vi "LAST 2.vi"() -> ()   [LabVIEW 2020]
uses:
  <vilib>/Instr/_visa.llb/VISA Configure Serial Port (Instr).vi
  <vilib>/measure/matone.llb/Extract Single Tone Information N Chan.vi
  <vilib>/measure/NI_MAPro.lvlib
panel:
  out "Filtered":dynamicdata(graph)
  out ".not. x?":bool
  out "?":dbl format="%#_4g"
  out "?":bool
  out "Gas level":dbl(knob) scale=0.0..2.0
  out "Buzzer":bool
  out "?":bool
  out "?":dbl
  out "Capacitor temperature":dbl(knob) scale=0.0..50.0
  out "Corrected Power Factor":dbl format="%#_4g"
  out "Active power(P)":dbl
  out "Reactive power(Q)":dbl
  out "Apperant power (S)":dbl
  out "Cap B":bool
  out "Cap A":bool
  out "Load Power Factor":dbl format="%#_4g"
  out "Calibearted\nPhase Angle (Radians)":dbl
  out "Calibearted\nPhase Angle (degrees)":dbl
  out "Real \nphase angle":dbl
  out "Current \nphase angle":dbl
  out "Voltage \nphase angle":dbl
  out "Cooling fan":bool
  in  "Virtual phase angle shifter":dbl(slide) scale=0.0..50.0
  in  "VISA resource name":refnum<visa-resource-name>
  in  "baud rate (9600)":u32=9600
  in  "Stop":bool
  # "Smart APFC Panel Control Dashboard"
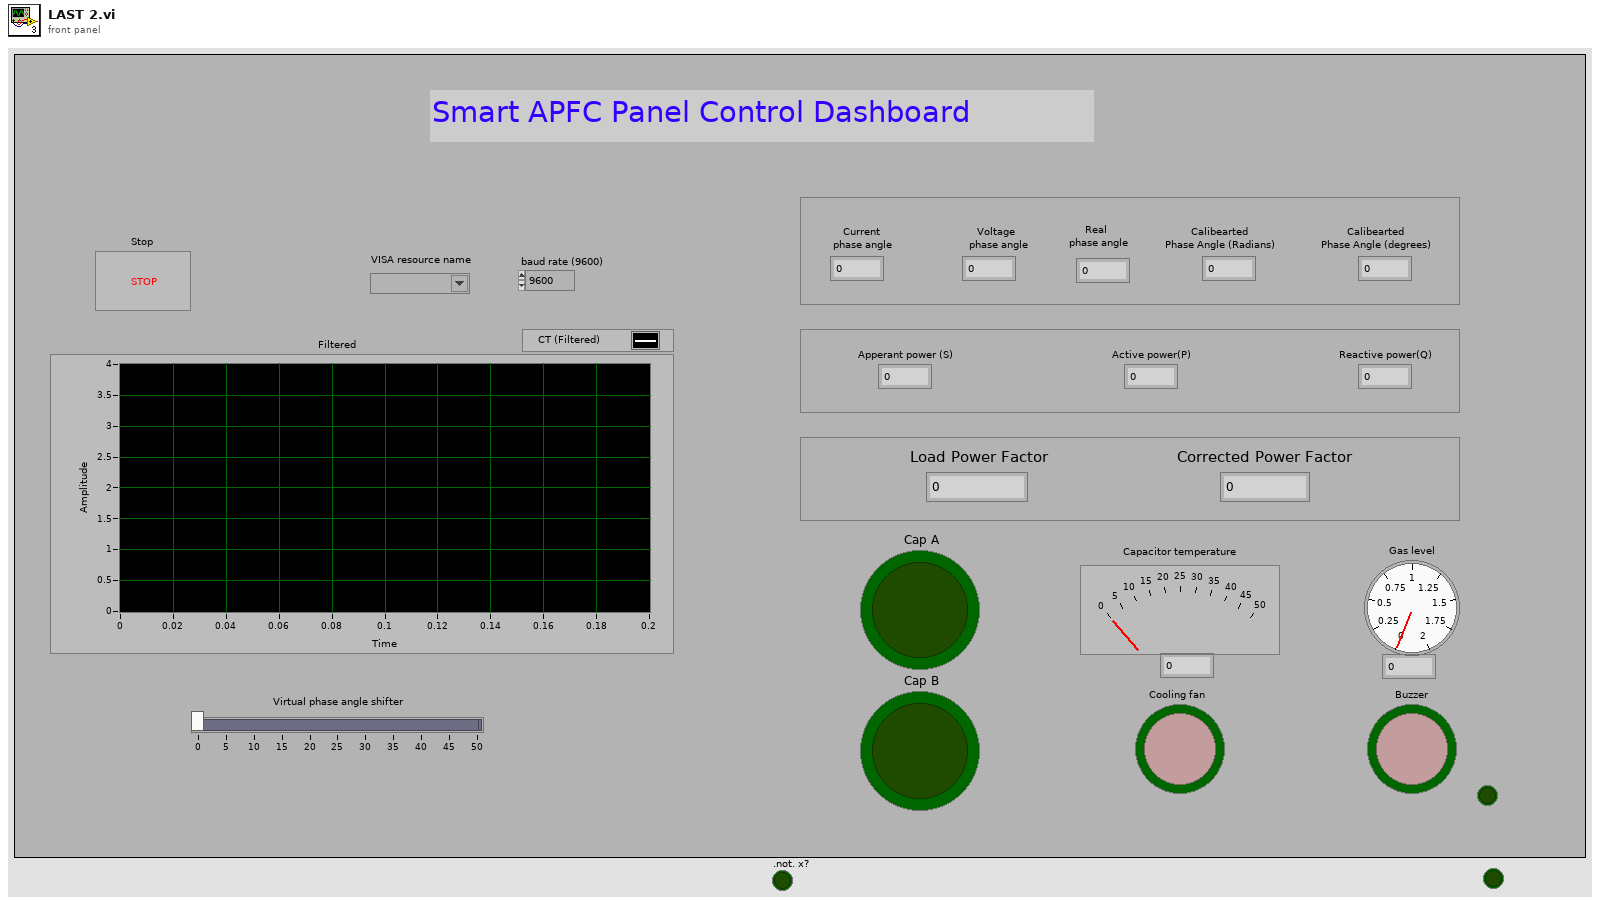
[diagram p1: front panel]
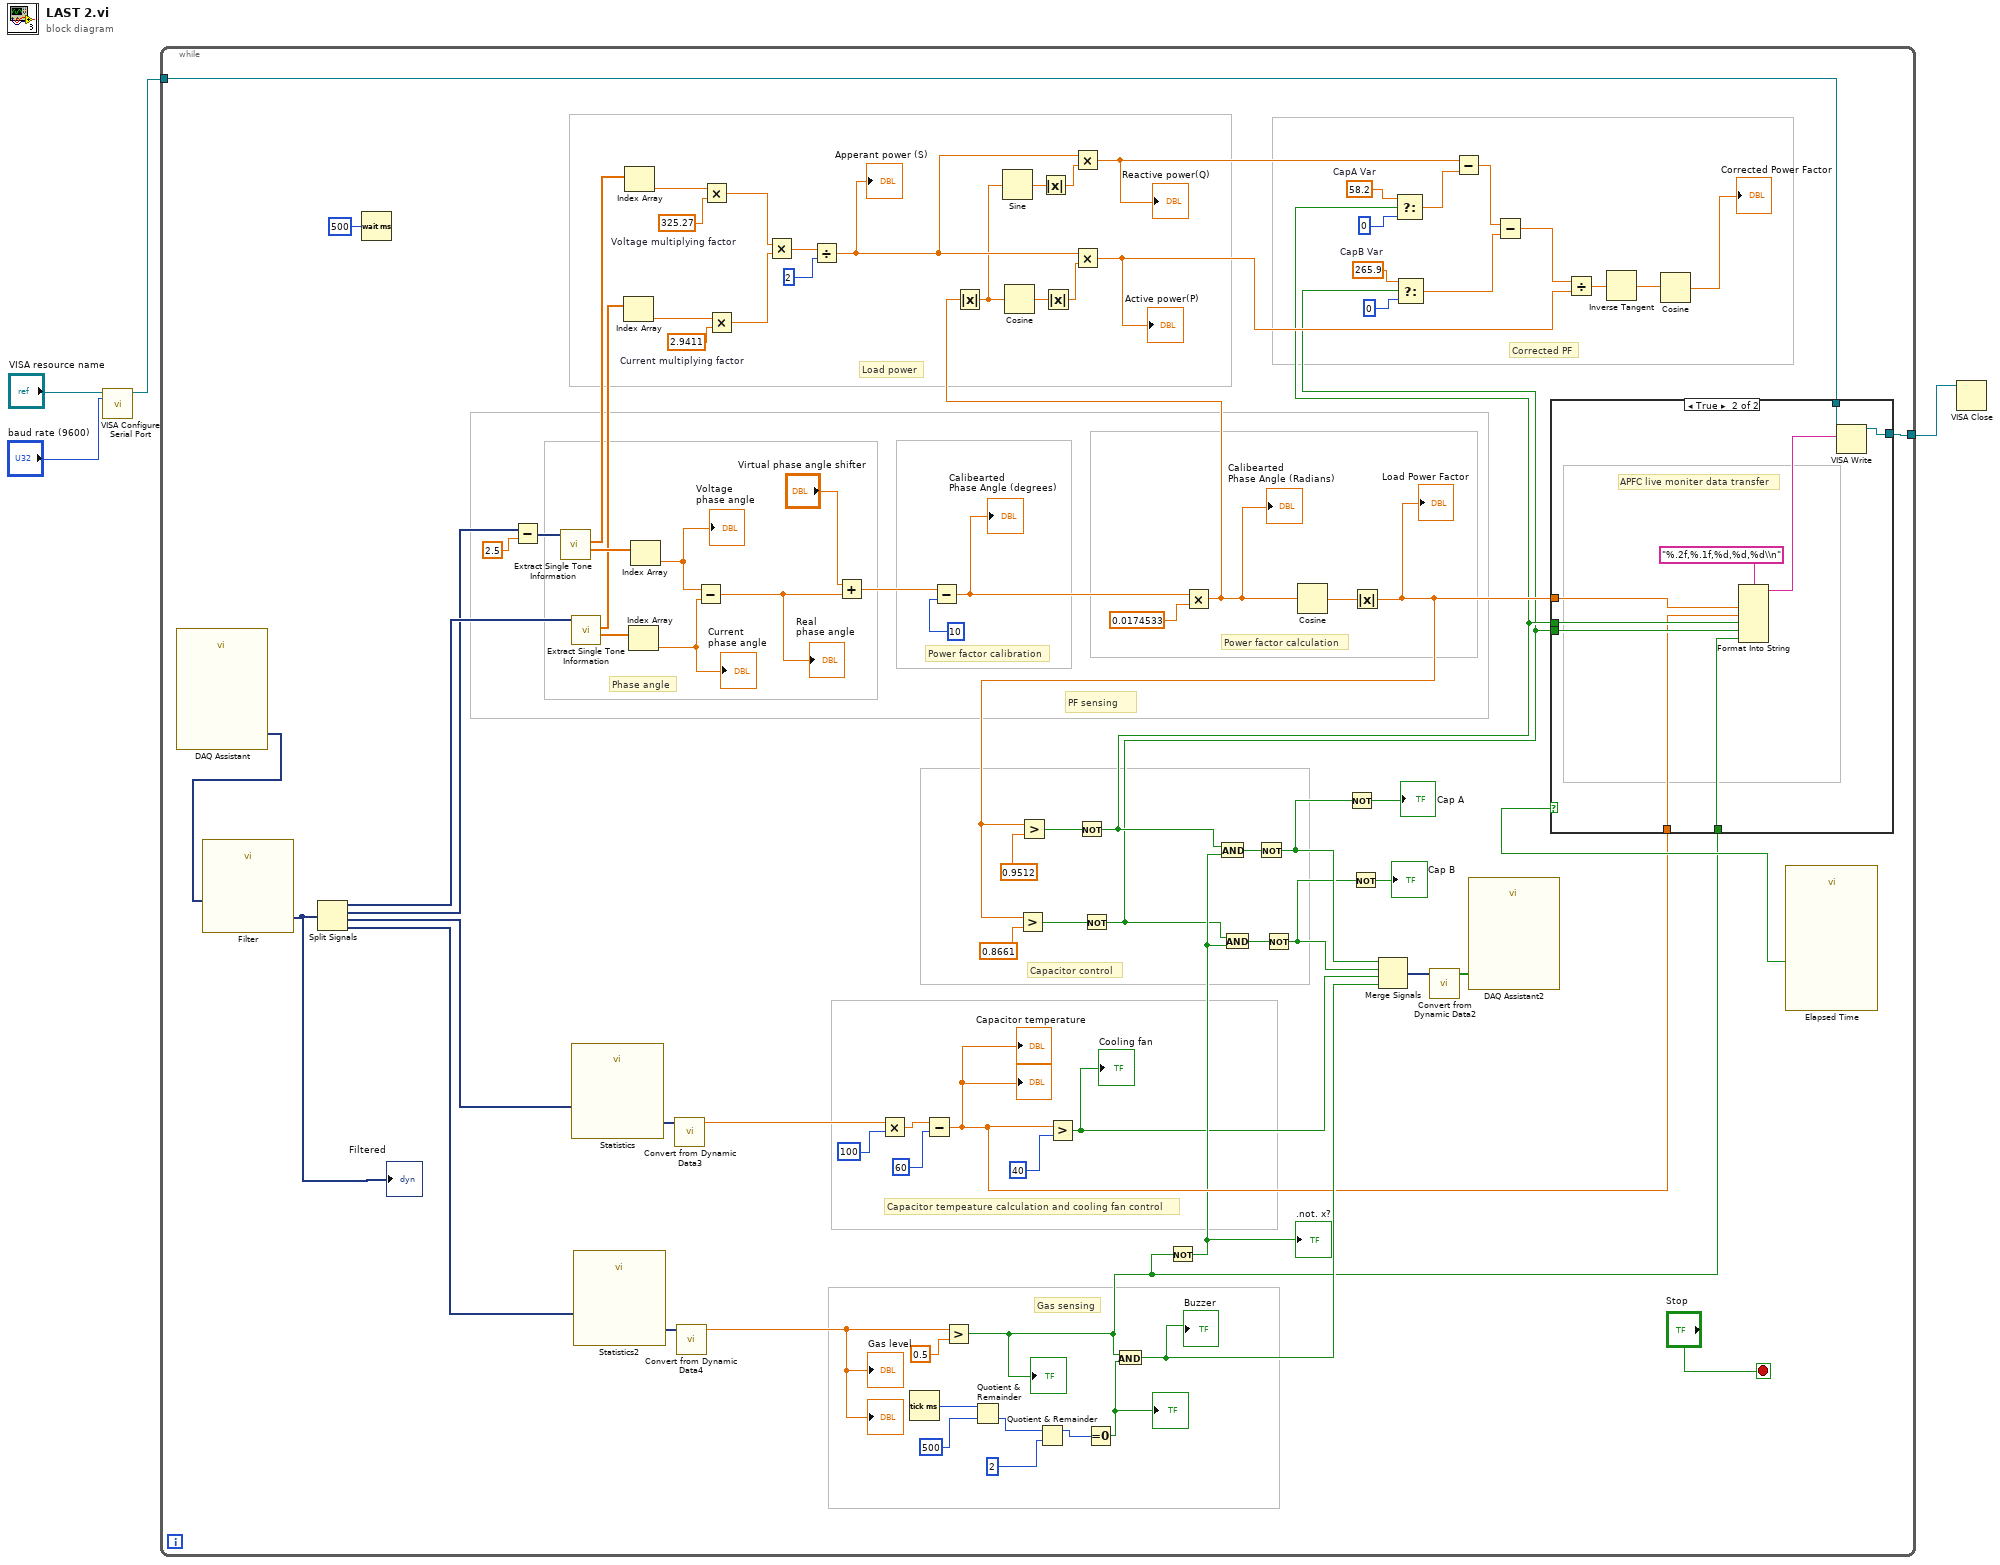
[diagram p0: block diagram]
diagram:
  n1 = call-poly "VISA Configure Serial Port"("VISA resource name"="VISA resource name", "baud rate (9600)"="baud rate (9600)") -> ("VISA resource name out"=w1:refnum<visa-resource-name>)  [unwired: 12 in, 1 out]
  n2 = while {
    tunnel: [w30] -> w4
    tunnel: w1 -> [w77]
    stop <- "Stop" stop-if-true
    w53 = 265.9  # CapB Var
    w54 = 58.2  # CapA Var
    w71 = 2.9411  # Current multiplying factor
    w72 = 325.27  # Voltage multiplying factor
    # "Corrected PF"
    # "Load power"
    # "PF sensing"
    # "Gas sensing"
    # "Power factor calibration"
    # "Capacitor tempeature calculation and cooling fan control"
    # "Power factor calculation"
    # "Phase angle"
    # "Capacitor control"
    n3 = call "DAQ Assistant"() -> ("data"=w5:dynamicdata)  [unwired: 17 in, 2 out]
    n4 = call "Filter"("Signal"=w5) -> ("Filtered Signal"=w6:dynamicdata)  [unwired: 9 in, 1 out]
    "Filtered" <- w6
    n5 = Split Signals(w6) -> (w92:dynamicdata, w83:dynamicdata, w74:dynamicdata, w40:dynamicdata)  [unwired: 4 in]
    n6 = Wait (ms)(milliseconds to wait=u32 500) -> ()  [unwired: 1 out]
    n7 = Subtract(x=w83, y=2.5) -> (x-y=w7:dynamicdata)
    n8 = call-poly <vilib>:"Extract Single Tone Information.vi"("time signals in"=w7) -> ("detected phases (deg)"=w63:dbl[], "detected amplitudes"=w58:dbl[])  [unwired: 5 in, 4 out]
    n9 = call-poly <vilib>:"Extract Single Tone Information.vi"("time signals in"=w92) -> ("detected phases (deg)"=w61:dbl[], "detected amplitudes"=w56:dbl[])  [unwired: 5 in, 4 out]
    n10 = call "Statistics"("Signals"=w74) -> ("Arithmetic Mean"=w75:dynamicdata)  [unwired: 25 in, 1 out]
    n11 = call "Statistics2"("Signals"=w40) -> ("Arithmetic Mean"=w41:dynamicdata)  [unwired: 25 in, 1 out]
    n12 = Index Array(array=w56) -> (element=w55:dbl)  [unwired: 1 in]
    n13 = Index Array(array=w58) -> (element=w57:dbl)  [unwired: 1 in]
    n14 = Index Array(array=w61) -> (element=w60:dbl)  [unwired: 1 in]
    "Current \nphase angle" <- w60
    n15 = Index Array(array=w63) -> (element=w62:dbl)  [unwired: 1 in]
    "Voltage \nphase angle" <- w62
    n16 = call "Convert from Dynamic Data3"("Dynamic Data Type"=w75) -> ("Scalar"=w73:dbl)  [unwired: 3 in]
    n17 = call "Convert from Dynamic Data4"("Dynamic Data Type"=w41) -> ("Scalar"=w29:dbl)  [unwired: 3 in]
    "Gas level" <- w29
    "?" <- w29
    n18 = Subtract(x=w62, y=w60) -> (x-y=w76:dbl)
    "Real \nphase angle" <- w76
    n19 = Multiply(x=w57, y=w72) -> (x*y=w70:dbl)
    n20 = Multiply(x=w55, y=w71) -> (x*y=w69:dbl)
    n21 = Multiply(x=w70, y=w69) -> (x*y=w68:dbl)
    n22 = Divide(x=w68, y=2) -> (x/y=w65:dbl)
    "Apperant power (S)" <- w65
    n23 = Add(x="Virtual phase angle shifter", y=w76) -> (x+y=w81:dbl)
    n24 = Multiply(x=w73, y=100) -> (x*y=w22:dbl)
    n25 = Tick Count (ms)() -> (millisecond timer value=w38:u32)
    n26 = Subtract(x=w22, y=60) -> (x-y=w23:dbl)
    "Capacitor temperature" <- w23
    "?" <- w23
    n27 = Subtract(x=w81, y=10) -> (x-y=w59:dbl)
    "Calibearted\nPhase Angle (degrees)" <- w59
    n28 = Greater?(x=w29, y=0.5) -> (0:w20:bool)
    "?" <- w20
    n29 = Quotient & Remainder(x=w38, y=500) -> (floor(x/y)=w35:u32)  [unwired: 1 out]
    n30 = Quotient & Remainder(x=w35, y=2) -> (x-y*floor(x/y)=w34:u32)  [unwired: 1 out]
    n31 = Greater?(x=w23, y=40) -> (0:w12:bool)
    "Cooling fan" <- w12
    n32 = Equal To 0?(x=w34) -> (x = 0?=w33:bool)
    "?" <- w33
    n33 = And(x=w20, y=w33) -> (x .and. y?=w32:bool)
    "Buzzer" <- w32
    n34 = Not(x=w20) -> (.not. x?=w16:bool)
    ".not. x?" <- w16
    n35 = Multiply(x=w59, y=0.0174533) -> (x*y=w66:dbl)
    "Calibearted\nPhase Angle (Radians)" <- w66
    n36 = Absolute Value(x=w66) -> (abs(x)=w64:dbl)
    n37 = Sine(x=w64) -> (sin(x)=w28:dbl)
    n38 = Cosine(x=w64) -> (cos(x)=w26:dbl)
    n39 = Absolute Value(x=w28) -> (abs(x)=w27:dbl)
    n40 = Absolute Value(x=w26) -> (abs(x)=w25:dbl)
    n41 = Multiply(x=w65, y=w27) -> (x*y=w50:dbl)
    "Reactive power(Q)" <- w50
    n42 = Multiply(x=w65, y=w25) -> (x*y=w42:dbl)
    "Active power(P)" <- w42
    n43 = Cosine(x=w66) -> (cos(x)=w84:dbl)
    n44 = Absolute Value(x=w84) -> (abs(x)=w24:dbl)
    "Load Power Factor" <- w24
    n45 = Greater?(x=w24, y=0.8661) -> (0:w14:bool)
    n46 = Greater?(x=w24, y=0.9512) -> (0:w18:bool)
    n47 = Not(x=w18) -> (.not. x?=w17:bool)
    n48 = Not(x=w14) -> (.not. x?=w13:bool)
    n49 = And(x=w17, y=w16) -> (x .and. y?=w19:bool)
    n50 = And(x=w13, y=w16) -> (x .and. y?=w15:bool)
    n51 = Not(x=w19) -> (.not. x?=w10:bool)
    n52 = Not(x=w15) -> (.not. x?=w8:bool)
    n53 = Not(x=w10) -> (.not. x?=→"Cap A":bool)
    n54 = Not(x=w8) -> (.not. x?=→"Cap B":bool)
    n55 = Merge Signals(w10, w8, w12, w32) -> (w88:dynamicdata)
    n56 = Select(t=w54, s=w17, f=0) -> (s? t:f=w49:dbl)
    n57 = Select(t=w53, s=w13, f=0) -> (s? t:f=w47:dbl)
    n58 = call "Convert from Dynamic Data2"("Dynamic Data Type"=w88) -> ("Array"=w87:bool[])  [unwired: 3 in]
    n59 = Subtract(x=w50, y=w49) -> (x-y=w48:dbl)
    n60 = call "DAQ Assistant2"("data"=w87) -> ()  [unwired: 17 in, 2 out]
    n61 = Subtract(x=w48, y=w47) -> (x-y=w43:dbl)
    n62 = Divide(x=w43, y=w42) -> (x/y=w46:dbl)
    n63 = Inverse Tangent(1:w46) -> (0:w45:dbl)
    n64 = Cosine(x=w45) -> (cos(x)=→"Corrected Power Factor":dbl)
    n65 = call "Elapsed Time"() -> ("Time has Elapsed"=w31:bool)  [unwired: 12 in, 7 out]
    n66 = case shown="True" w31 {
      tunnel: [w94 w101] -> w30
      tunnel: w77 -> [w94 w100]
      tunnel: w24 -> [_ w99]
      tunnel: w17 -> [_ w98]
      tunnel: w13 -> [_ w97]
      tunnel: w23 -> [_ w96]
      tunnel: w20 -> [_ w95]
      frame False {
      }
      frame True {
        # "APFC live moniter data transfer"
        n67 = Format Into String(format string="%.2f,%.1f,%d,%d,%d\\n", w99, w96, w98, w97, w95) -> (resulting string=w102:string)  [unwired: 2 in, 1 out]
        n68 = VISA Write(VISA resource name=w100, write buffer=w102) -> (VISA resource name out=w101:refnum<visa-resource-name>)  [unwired: 1 in, 2 out]
      }
    }
  }
  n69 = VISA Close(VISA resource name=w4) -> ()  [unwired: 1 in, 1 out]
